vi "image_acquisition.vi"(9 "Input\nparameters":T2={"Frame rate (ms)"=2000, "Worm Strain"="N2", "Time t"=0, "State"=enum."Image acquisition", "Acquisition time"=0.0, "Maximum # of images"=100000, "#TTL"=0, "time of third ttl "=100000, "ImSub Value"=0, "Time of last TTL"=0, "# Rows"=2, "# Columns"=2, "number of adjacentTTL"=0, "Sleep Deprivation status"="", "Sleep Detection"=FALSE, "Time of first sleep detection"=0, "# Sleep detections"=0, "Time max # adjacent TTL"=-10000, "Image t-1"=[], "Image t"=[]} {"# Columns" items=["1"=1, "2"=2, "3"=3, "4"=4]; "# Rows" items=["1"=1, "2"=2, "3"=3, "4"=4]}, 10 "Display\nImage":bool, 11 "Frame\nrate (ms)":u32=2000) -> (1 "Output\nparameters":T2={"Frame rate (ms)"=2000, "Worm Strain"="N2", "Time t"=0, "State"=enum."Image acquisition", "Acquisition time"=0.0, "Maximum # of images"=100000, "#TTL"=0, "time of third ttl "=100000, "ImSub Value"=0, "Time of last TTL"=0, "# Rows"=2, "# Columns"=2, "number of adjacentTTL"=0, "Sleep Deprivation status"="", "Sleep Detection"=FALSE, "Time of first sleep detection"=0, "# Sleep detections"=0, "Time max # adjacent TTL"=-10000, "Image t-1"=[], "Image t"=[]} {"# Columns" items=["1"=1, "2"=2, "3"=3, "4"=4]; "# Rows" items=["1"=1, "2"=2, "3"=3, "4"=4]}, 2 "Acquisition\nsuccessfull":bool, 3 "Intensity Graph 2":u16[][](graph))   [LabVIEW 2011]
uses:
  state.ctl
panel:
  # "General settings"
  # "Select number of animals"
  # "Row"
  # "Column"
  # "General settings"
  # "Select number of animals"
  # "Row"
  # "Column"
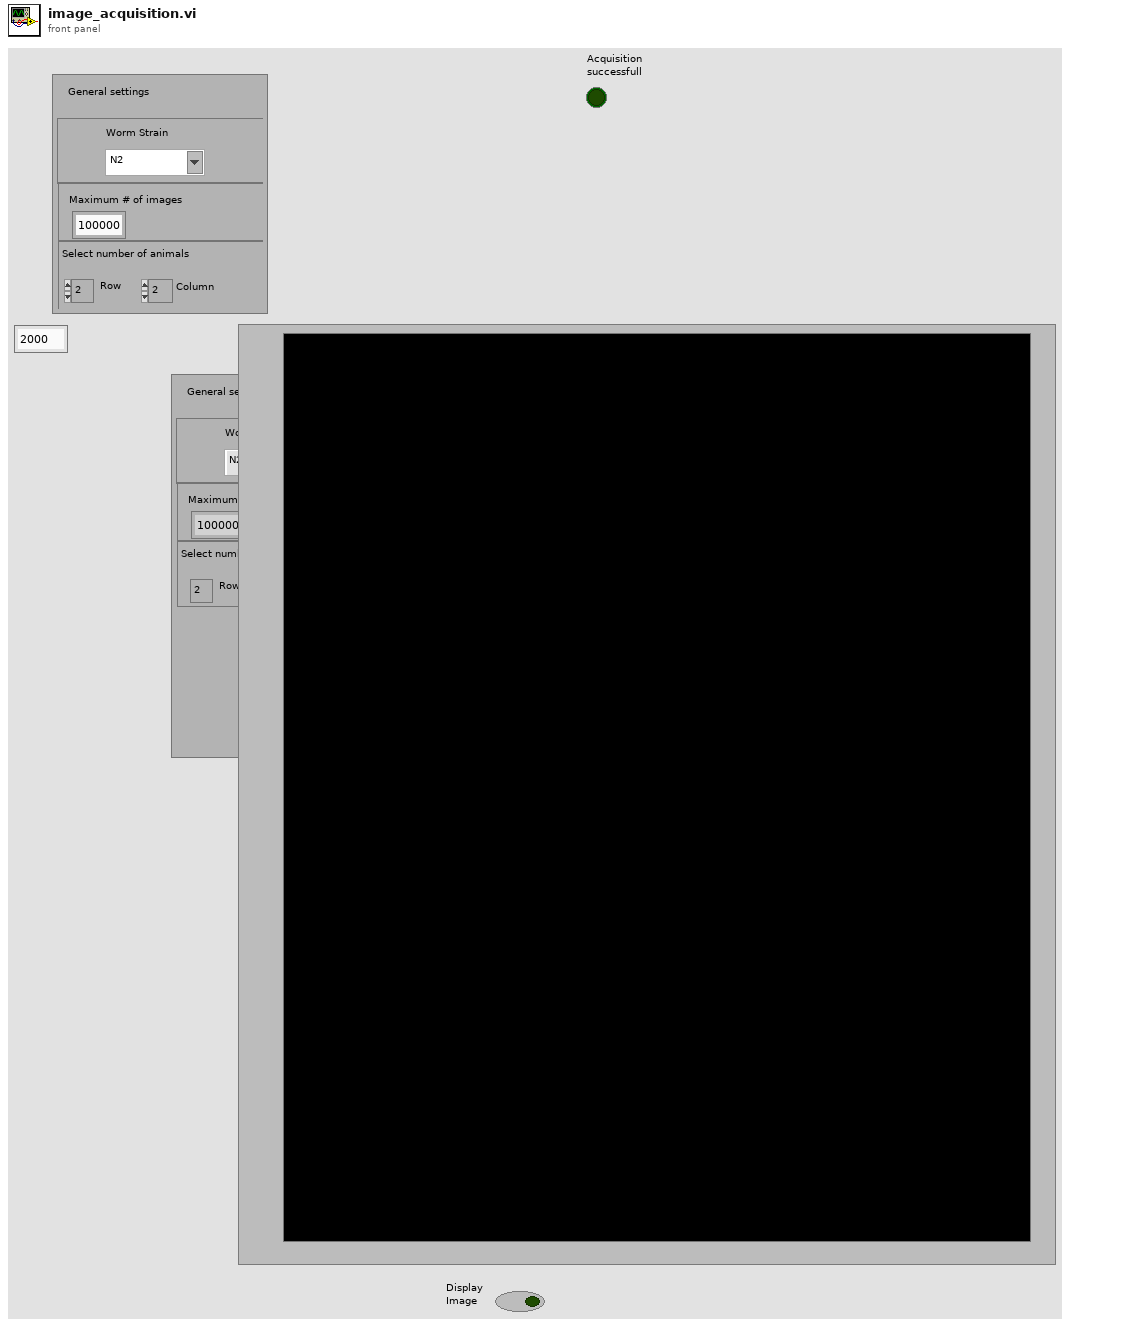
[diagram p1: front panel]
types:
  T1 = typedef "state.ctl" = enum16{"Initialize measurement", "Image acquisition", "Image processing", "Sleep detection", "Control TTL protocol ", "Sleep deprivation", "Update image & exit condition", "Wait "}
  T2 = cluster{"Frame rate (ms)":u32, "Worm Strain":string, "Time t":i32, "State":T1, "Acquisition time":dbl, "Maximum # of images":i32, "#TTL":i32, "time of third ttl ":i32, "ImSub Value":i32, "Time of last TTL":i32, "# Rows":u32, "# Columns":u32, "number of adjacentTTL":i32, "Sleep Deprivation status":string, "Sleep Detection":bool, "Time of first sleep detection":i32, "# Sleep detections":i32, "Time max # adjacent TTL":i32, "Image t-1":i32[][], "Image t":i32[][]}
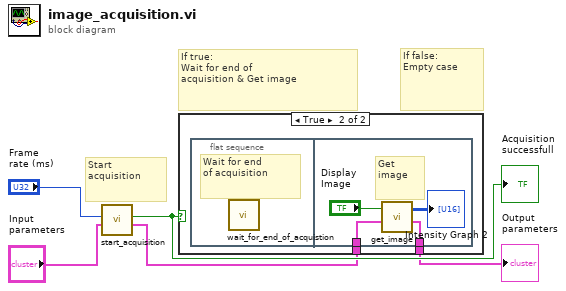
[diagram p0: block diagram]
diagram:
  # "If true:\nWait for end of\nacquisition & Get image"
  # "If false:\nEmpty case"
  # "Start\nacquisition"
  n1 = call "start_acquisition.vi"("Input\nparameters"="Input\nparameters", "Frame rate"="Frame\nrate (ms)") -> ("Output\nparameters"=w2:T2, "Acquisition\nsuccessfull"=w4:bool)  [unwired: 8 in]
  "Acquisition\nsuccessfull" <- w4
  n2 = case shown="True" w4 {
    tunnel: w2 -> [w6 w8]
    tunnel: [w6 w7] -> w1
    frame False {
    }
    frame True {
      n3 = flat-sequence {
        tunnel: w8 -> [w10]
        tunnel: [w9] -> w7
        frame #0 {
          # "Wait for end\nof acquisition"
          n4 = call "wait_for_end_of_acquistion.vi"() -> ()  [unwired: 12 in]
        }
        frame #1 {
          # "Get\nimage"
          n5 = call "get_image.vi"("Input\nparameters"=w10, 10:"Display\nImage") -> ("Output\nparameters"=w9:T2, "Intensity Graph"=→"Intensity Graph 2":u16[][])  [unwired: 8 in]
        }
      }
    }
  }
  "Output\nparameters" <- w1
